vi "1WIRE_Write_Bit.vi"(7 "1-Wire DIO Pin":refnum<k21>="ConnectorA/DIO15", 8 "Error In":errorcluster, 10 "Bit":bool) -> (0 "Error Out":errorcluster)   [LabVIEW 2014]
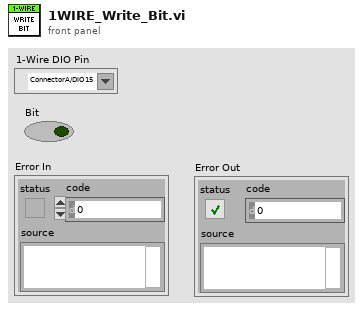
[diagram p1: front panel]
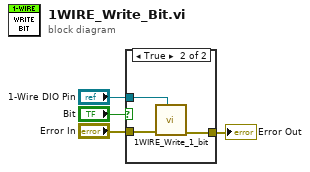
[diagram p0: block diagram]
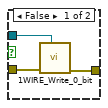
[diagram p2: hidden frame]
diagram:
  n1 = case shown="True" "Bit" {
    tunnel: "1-Wire DIO Pin" -> [w5 w10]
    tunnel: "Error In" -> [w7 w9]
    tunnel: [w6 w8] -> w1
    frame False {
      n2 = call "1WIRE_Write_0_bit.vi"("1-Wire DIO Pin"=w5, "error in"=w7) -> ("error out"=w6:errorcluster)  [unwired: 9 in]
    }
    frame True {
      n3 = call "1WIRE_Write_1_bit.vi"("1-Wire DIO Pin"=w10, "error in"=w9) -> ("error out"=w8:errorcluster)  [unwired: 9 in]
    }
  }
  "Error Out" <- w1
